vi "iNi.xio.vi"(5 "configuration file path":path, 6 "Sections":string, 7 "error in (no error)":errorcluster caption="错误输入（无错误）") -> (0 "configuration file path":path, 1 "TagsOut":cluster{"Tags":string, "Value":string}[](array[cluster]), 2 "Values":string[](array[string]), 3 "error out":errorcluster caption="错误输出", 4 "Count":i32[](array[numeric]))   [LabVIEW 2018]
uses:
  <vilib>/Utility/config.llb/Read Key (String).vi
  <vilib>/Utility/config.llb/NI_LVConfig.lvlib
panel:
  # "General"
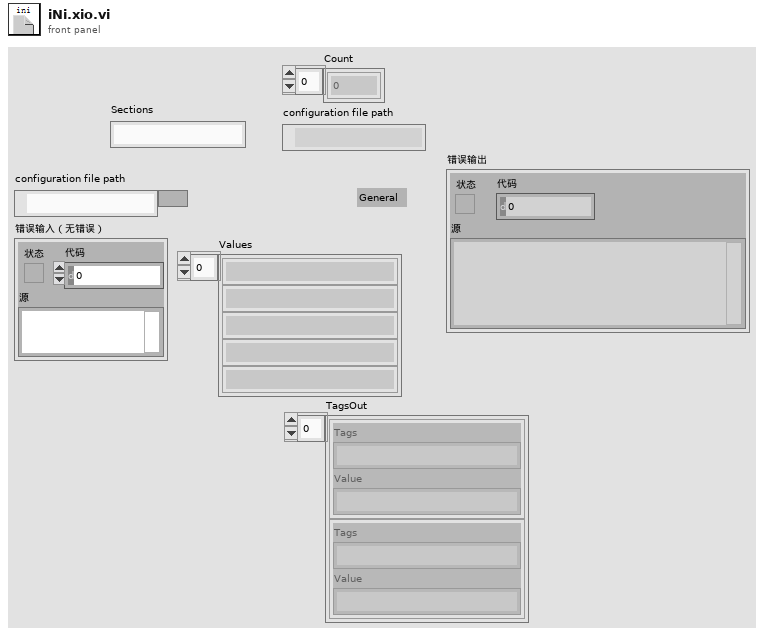
[diagram p1: front panel]
types:
  T1 = typedef "NI_LVConfig.lvlib/Config Data RefNum.ctl" = refnum<k1>
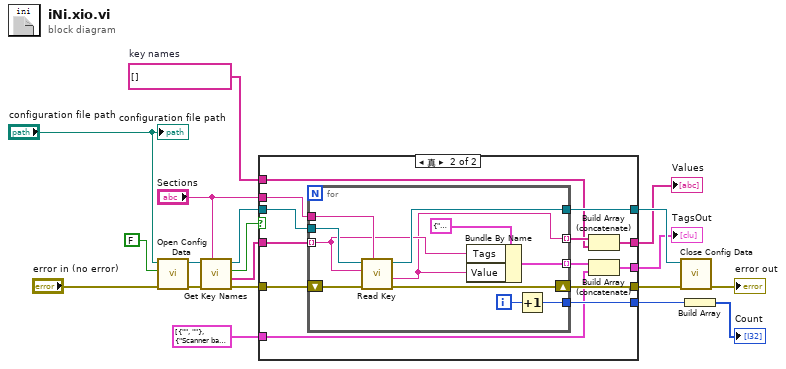
[diagram p0: block diagram]
diagram:
  w10 = string[] []  # key names
  n1 = call <vilib>:"Open Config Data.vi"("error in (no error)"="error in (no error)", "create file if necessary (T)"=FALSE, "configuration file path"="configuration file path") -> ("error out"=w15:errorcluster, "refnum"=w16:T1)  [unwired: 6 in, 1 out]
  n2 = call <vilib>:"Get Key Names.vi"("section"="Sections", "error in (no error)"=w15, "refnum"=w16) -> ("error out"=w4:errorcluster, "key names"=w3:string[], "section exists?"=w6:bool, "refnum out"=w5:T1)  [unwired: 5 in]
  n3 = case shown="真" w6 {
    tunnel: w5 -> [w20 w35]
    tunnel: w4 -> [w21 w34]
    tunnel: w3 -> [w22 w33]
    tunnel: "Sections" -> [_ w32]
    tunnel: [w21 w31] -> w13
    tunnel: [w20 w30] -> w14
    tunnel: [w22 w28] -> w11
    tunnel: w10 -> [_ w27]
    tunnel: [_ w26] -> w2
    tunnel: cluster{"Tags":string, "Value":string}[] [{"Tags"="", "Value"=""}, {"Tags"="Scanner baud rate", "Value"="9600"}, {"Tags"="Scanner1 Com", "Value"="COM2"}, {"Tags"="Scanner2 Com", "Value"="COM3"}, {"Tags"="Scanner3 Com", "Value"=""}, {"Tags"="Scanner4 Com", "Value"=""}, {"Tags"="Scanner5 Com", "Value"=""}] ("TagsOut") -> [_ w25]
    tunnel: [_ w23] -> w8
    frame False {
    }
    frame True {
      n4 = for {
        tunnel: w35 -> [w46]
        tunnel: w33 -> [w38] mode=indexing
        tunnel: w32 -> [w44]
        shift-right: [w43] -> w31
        shift-left: w34 -> [w45]
        tunnel: [w37] -> w29 mode=indexing
        tunnel: [w42] -> w30
        tunnel: [w40] -> w26
        tunnel: [w36] -> w24 mode=indexing
        i -> [w41]
        n5 = call-poly <vilib>:"Read Key.vi"("section"=w44, "error in (no error)"=w45, "key"=w38, "refnum"=w46) -> ("error out"=w43:errorcluster, "value"=w37:string, "refnum out"=w42:T1)  [unwired: 4 in, 1 out]
        n6 = Bundle By Name(cluster=cluster{"Tags":string, "Value":string} {"Tags"="", "Value"=""}, "Tags"=w38, "Value"=w37) -> (w36:cluster{"Tags":string, "Value":string})
        n7 = Increment(x=w41) -> (x+1=w40:i32)
      }
      n8 = Build Array (concatenate)(w29, w27) -> (w28:string[])
      n9 = Build Array (concatenate)(w24, w25) -> (w23:cluster{"Tags":string, "Value":string}[])
    }
  }
  "Values" <- w11
  "TagsOut" <- w8
  n10 = call <vilib>:"Close Config Data.vi"("error in (no error)"=w13, "refnum"=w14) -> ("error out"=→"error out":errorcluster)  [unwired: 8 in, 1 out]
  n11 = Build Array(w2) -> (→"Count":i32[])
  "configuration file path" <- "configuration file path"
